vi "Graph Initialize Y scale.vi"(8 "error in (no error)":errorcluster, 9 "Y scale":T1, 10 "Active Y Scale":i32, 11 "Chart Ref":refnum<vi>) -> (0 "error out":errorcluster)   [LabVIEW 2011]
uses:
  Y scale cluster.ctl
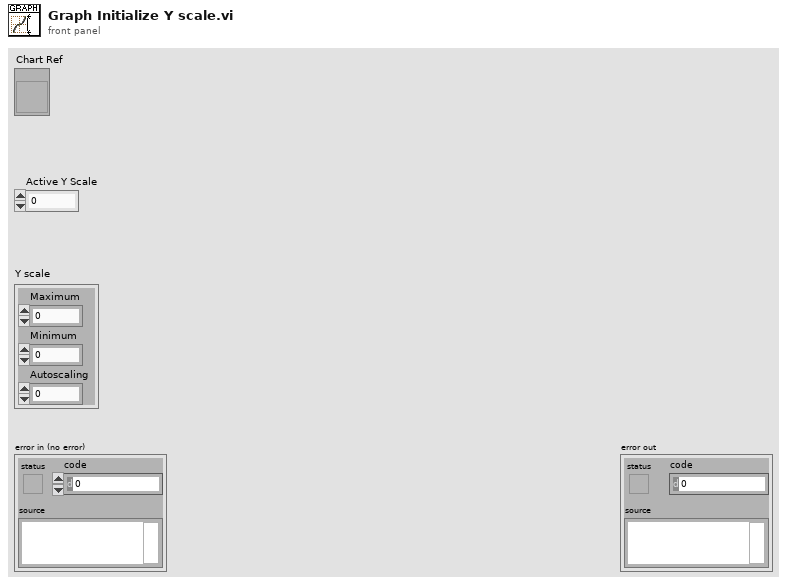
[diagram p1: front panel]
types:
  T1 = typedef "Y scale cluster.ctl" = cluster{"Maximum":dbl, "Minimum":dbl, "Autoscaling":i32}
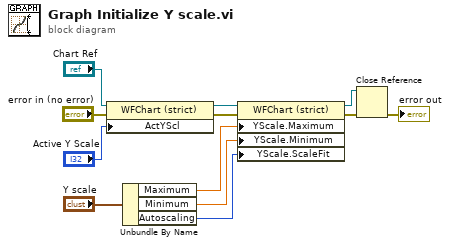
[diagram p0: block diagram]
diagram:
  n1 = property class="WFChart (strict)"(reference="Chart Ref", error in="error in (no error)", "ActYScl"="Active Y Scale") -> (reference out=w12:refnum<vi>, error out=w7:errorcluster)
  n2 = Unbundle By Name("Y scale") -> ("Maximum"=w10:dbl, "Minimum"=w9:dbl, "Autoscaling"=w8:i32)
  n3 = property class="WFChart (strict)"(reference=w12, error in=w7, "YScale.Maximum"=w10, "YScale.Minimum"=w9, "YScale.ScaleFit"=w8) -> (reference out=w3:refnum<vi>, error out=w2:errorcluster)
  n4 = Close Reference(reference=w3, error in (no error)=w2) -> (error out=→"error out":errorcluster)
